vi "pH,SO2,temp formulas (SubVI).vi"(8 "Numeric 7":u16, 9 "Numeric 4":u16, 10 "Numeric in":u16, 11 "Numeric 6":u16) -> (1 "Numeric 3":dbl, 2 "Numeric 5":dbl, 3 "Numeric out":dbl)   [LabVIEW 2016]
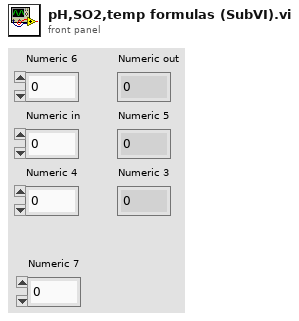
[diagram p1: front panel]
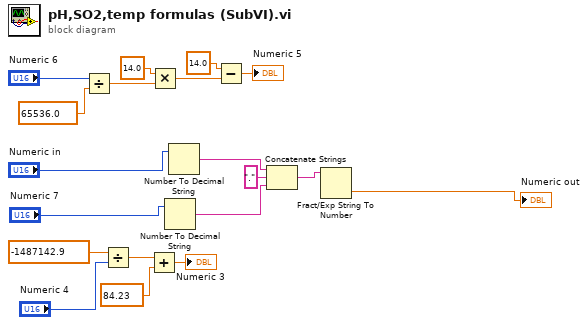
[diagram p0: block diagram]
diagram:
  n1 = Divide(x="Numeric 6", y=65536.0) -> (x/y=w10:dbl)
  n2 = Divide(x=-1487142.9, y="Numeric 4") -> (x/y=w17:dbl)
  n3 = Add(x=w17, y=84.23) -> (x+y=→"Numeric 3":dbl)
  n4 = Multiply(x=14.0, y=w10) -> (x*y=w12:dbl)
  n5 = Number To Decimal String(number="Numeric 7") -> (decimal integer string=w4:string)  [unwired: 1 in]
  n6 = Number To Decimal String(number="Numeric in") -> (decimal integer string=w5:string)  [unwired: 1 in]
  n7 = Subtract(x=14.0, y=w12) -> (x-y=→"Numeric 5":dbl)
  n8 = Concatenate Strings(w5, "." ("string"), w4) -> (w2:string)
  n9 = Fract/Exp String To Number(string=w2) -> (number=→"Numeric out":dbl)  [unwired: 3 in, 1 out]
